vi "Set Signal Manager.vi"(0 "Tosca in":refnum<class "Parameters.lvclass">, 5 "stateIndex":i32, 7 "SigMan":refnum<class "SignalManager.lvclass">, 11 "error in (no error)":errorcluster) -> (4 "Tosca out":refnum<class "Parameters.lvclass">, 15 "error out":errorcluster)   [LabVIEW 2020, in "Parameters.lvclass"]
uses:
  Parameters.lvclass
  epl-vi-lib/Signal Synthesis VIs/4th Generation/Classes/SignalManager/SignalManager.lvclass
  Parameters.lvclass/Parameters.ctl
  State/State.lvclass/State.ctl
  State/Write SigMan.vi
  State/State.lvclass
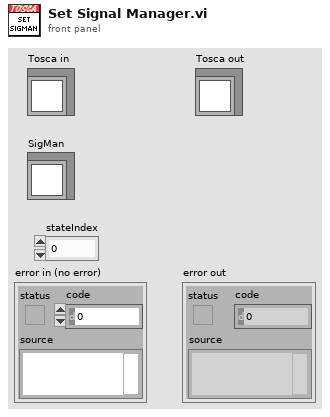
[diagram p1: front panel]
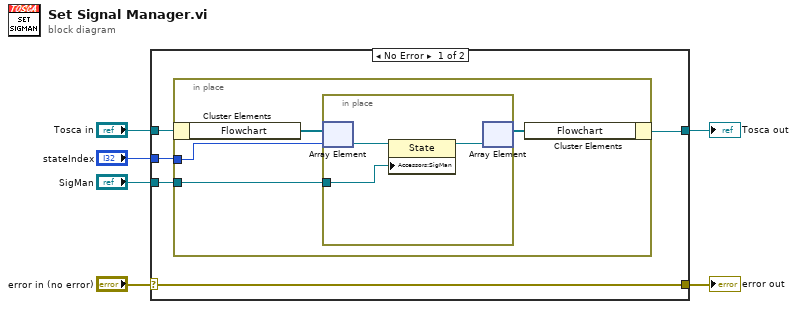
[diagram p0: block diagram]
diagram:
  n1 = case shown="No Error" "error in (no error)" {
    selector: "error in (no error)" -> [w11 w20]
    tunnel: [w11 w20] -> w5
    tunnel: [w7 w19] -> w3
    tunnel: "Tosca in" -> [w10 w19]
    tunnel: "stateIndex" -> [w9 _]
    tunnel: "SigMan" -> [w8 _]
    frame No Error {
      n2 = in-place {
        in-place-border: w9 -> [w14]
        in-place-border: w8 -> [w12]
        n3 = in-place-cluster #1(w10) -> ("Flowchart"=w15:refnum<class "State.lvclass">[])
        n4 = in-place {
          in-place-border: w12 -> [w16]
          n5 = in-place-array #2(w15, w14) -> (w18:refnum<class "State.lvclass">)
          n6 = property class="State"(reference=w18, "Accessors:SigMan"=w16) -> (reference out=w17:refnum<class "State.lvclass">)  [unwired: 1 in, 1 out]
          n7 = in-place-array #2(w17) -> (w13:refnum<class "State.lvclass">[])  [unwired: 1 out]
        }
        n8 = in-place-cluster #1("Flowchart"=w13) -> (w7:refnum<class "Parameters.lvclass">)
      }
    }
    frame Error {
    }
  }
  "error out" <- w5
  "Tosca out" <- w3
